vi "RT_Coriolis_Force_in_DLR_Navigation_Reference_System(SubVI).vi"(0 "Data":dbl[][](array[numeric]), 2 "le (m) in":dbl, 5 "i":i32, 9 "DCM":dbl[][](array[numeric]), 11 "W_b (rad/s)":dbl[](array[numeric])) -> (4 "Fco (N)":dbl[](array[numeric]))   [LabVIEW 2017]
uses:
  <vilib>/Analysis/baseanly.llb/Real A x B.vi
  <vilib>/Analysis/Matrix/Numeric/Conversions/Array To Matrix - RA.vi
  <vilib>/Analysis/Matrix/Numeric/Conversions/Array To Matrix - RA2.vi
  <vilib>/Analysis/Matrix/Numeric/Conversions/Matrix To Array - RM.vi
  <vilib>/Analysis/NI_AALBase.lvlib
  <vilib>/Analysis/Matrix/NI_Matrix.lvlib
  <vilib>/Analysis/NI_AALPro.lvlib
panel:
  out "OMEGA":dbl[](array[numeric])
  out "m":dbl
  out "Re":dbl[](array[numeric])
  out "re":dbl
  out "CoG (m)":dbl
  out "M_p (kg/s)":dbl
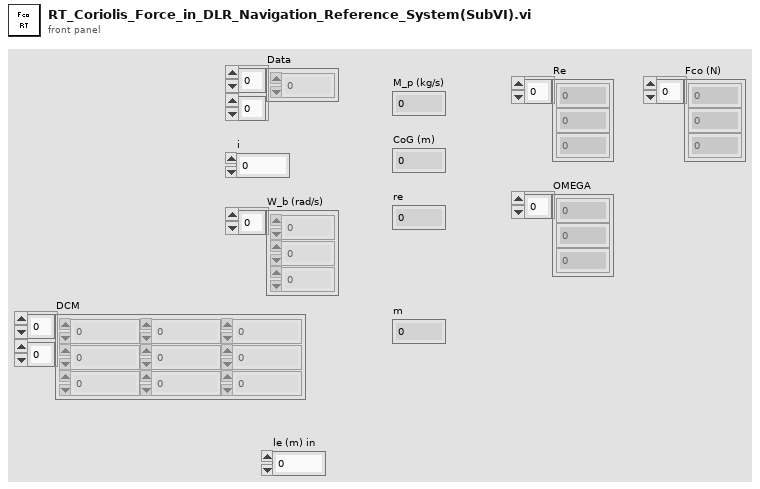
[diagram p1: front panel]
types:
  T1 = typedef "NI_Matrix.lvlib/RealMatrix.ctl" = dbl[][]
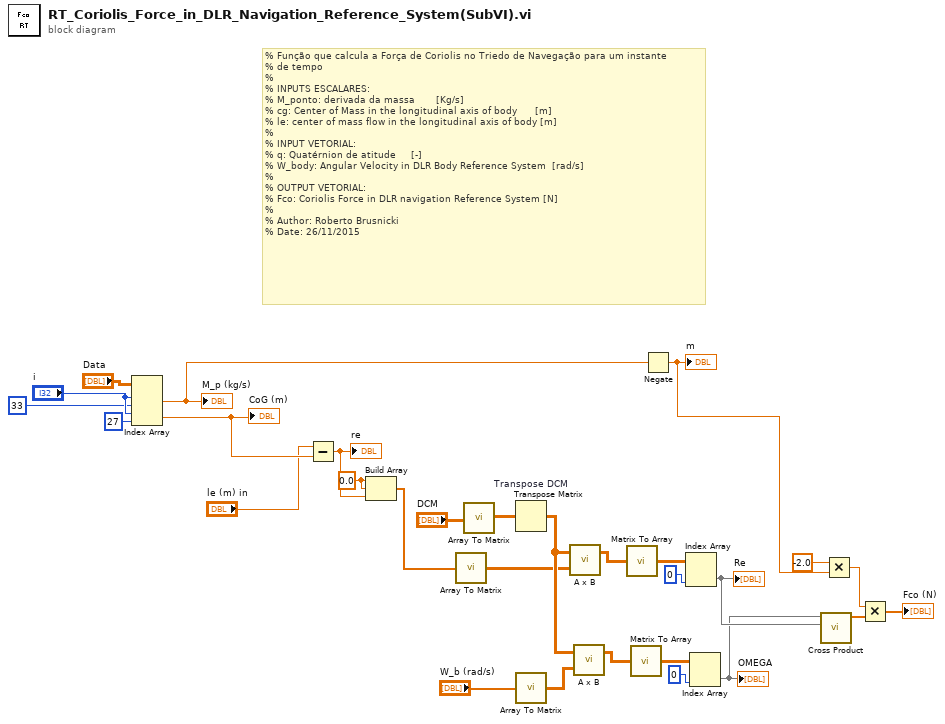
[diagram p0: block diagram]
diagram:
  w14 = 0.0 ("element")
  # "% Função que calcula a Força de Coriolis no Triedo de Navegação para um instante\n% de tempo\n%\n% INPUTS ESCALARES:\n% M_ponto: derivada da massa\t\t\t\t   [Kg/s]\n% cg: Center of Mass in the longitudinal axis of body      [m]\n% le: center of mass flow in the longitudinal axis of body [m]\n% \n% INPUT VETORIAL:\n% q: Quatérnion de atitude\t\t\t\t [-]\n% W_body: Angular Velocity in DLR Body Reference System  [rad/s] \t\n%\n% OUTPUT VETORIAL:\n% Fco: Coriolis Force in DLR navigation Reference System [N]\n%\n% Author: Roberto Brusnicki\n% Date: 26/11/2015"
  n1 = Index Array(array="Data", index (row) #1="i", index (col) #1=33 ("disabled index (col)"), index (row) #2="i", index (col) #2=27 ("disabled index (col)")) -> (element #1=w17:dbl, element #2=w9:dbl)
  "M_p (kg/s)" <- w17
  "CoG (m)" <- w9
  n2 = Subtract(x="le (m) in", y=w9) -> (x-y=w13:dbl)
  "re" <- w13
  n3 = Build Array(w14, w14, w13) -> (w15:dbl[])
  n4 = call-poly <vilib>:"Array To Matrix.vi"("Real 1D Array"=w15) -> ("Real Matrix (Column Vector)"=w12:T1)
  n5 = call-poly <vilib>:"Array To Matrix.vi"("Real 2D Array"="DCM") -> ("Real Matrix"=w16:T1)
  n6 = Transpose Matrix "Transpose DCM"(1:w16) -> (0:w21:T1)
  n7 = call-poly <vilib>:"Array To Matrix.vi"("Real 1D Array"="W_b (rad/s)") -> ("Real Matrix (Column Vector)"=w18:T1)
  n8 = call-poly <vilib>:"A x B.vi"("B"=w12, "A"=w21) -> ("A x B"=w10:T1)  [unwired: 1 out]
  n9 = call-poly <vilib>:"A x B.vi"("B"=w18, "A"=w21) -> ("A x B"=w20:T1)  [unwired: 1 out]
  n10 = call-poly <vilib>:"Matrix To Array.vi"("Real Matrix"=w10) -> ("Real 2D Array"=w11:dbl[][])
  n11 = call-poly <vilib>:"Matrix To Array.vi"("Real Matrix"=w20) -> ("Real 2D Array"=w19:dbl[][])
  n12 = Negate(x=w17) -> (-x=w25:dbl)
  "m" <- w25
  n13 = Index Array(array=w11, index (col)=0 ("index (row)")) -> (element=w24:dbl[])  [unwired: 1 in]
  "Re" <- w24
  n14 = Index Array(array=w19, index (col)=0 ("index (row)")) -> (element=w23:dbl[])  [unwired: 1 in]
  "OMEGA" <- w23
  n15 = call <vilib>:"Cross Product.vi"("B Vector"=w24, "A Vector"=w23) -> ("Cross Product"=w28:dbl[])  [unwired: 8 in, 1 out]
  n16 = Multiply(x=-2.0, y=w25) -> (x*y=w27:dbl)
  n17 = Multiply(x=w27, y=w28) -> (x*y=→"Fco (N)":dbl[])
